vi "Are Servers Connected.vi"(5 "Wait":bool=TRUE, 6 "Activity":string, 9 "error in":errorcluster) -> (0 "Connected?":bool, 3 "error out":errorcluster)   [LabVIEW 2013]
uses:
  _ROSDefinition.vi
panel:
  out "History":string
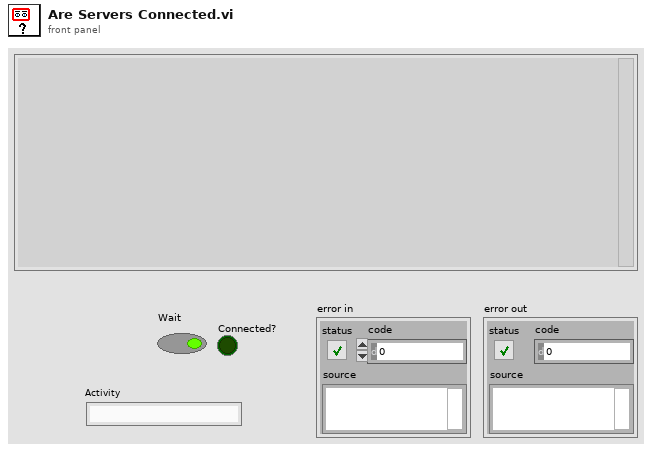
[diagram p1: front panel]
types:
  T1 = cluster{"server vi":string, "reference":refnum<vi>, "Description":string[], "Connected":bool}[]
  T2 = enum32{"Bad", "Idle", "Run top level", "Running"}
  T3 = cluster{"server vi":string, "reference":refnum<vi>, "Description":string[], "Connected":bool}
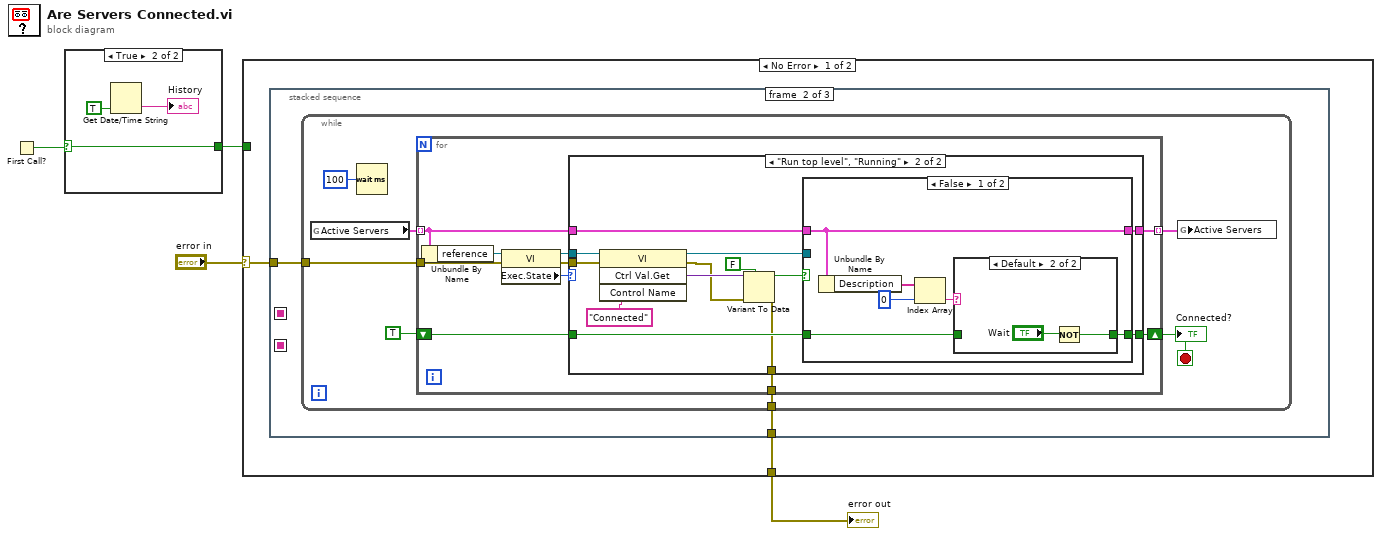
[diagram p0: block diagram]
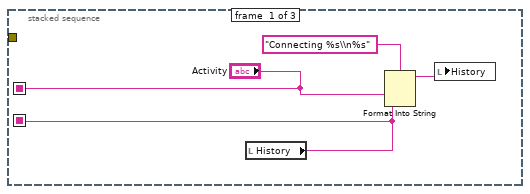
[diagram p3: hidden frame]
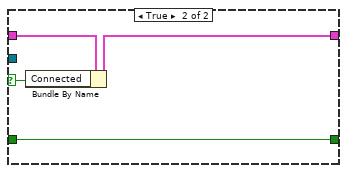
[diagram p6: hidden frame]
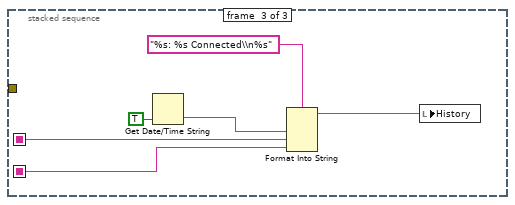
[diagram p7: hidden frame]
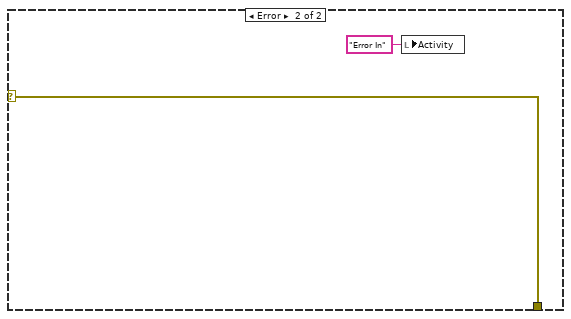
[diagram p8: hidden frame]
diagram:
  n1 = First Call?() -> (First Call?: T/F=w2:bool)
  n2 = case shown="True" w2 {
    selector: w2 -> [w5 w8]
    tunnel: [w5 w8] -> w1
    frame False {
    }
    frame True {
      n3 = Get Date/Time String(want seconds? (F)=TRUE) -> (time string=→"History":string)  [unwired: 2 in, 1 out]
    }
  }
  n4 = case shown="No Error" "error in" {
    selector: "error in" -> [w10 w70]
    tunnel: [w9 w70] -> w3
    tunnel: w1 -> [_ _]
    frame No Error {
      n5 = stacked-sequence {
        seq-local: ["Activity" _ _] -> [_ _ w65]
        seq-local: [w11 _ _] -> [_ _ w64]
        tunnel: w10 -> [_ w16 _]
        tunnel: [_ w15 _] -> w9
        frame #0 {
          n6 = local read "History"() -> (w11:string)
          n7 = Format Into String(format string="Connecting %s\\n%s", "Activity", w11) -> (resulting string=w12:string)  [unwired: 2 in, 1 out]
          n8 = local write "History"(w12) -> ()
        }
        frame #1 {
          n9 = while {
            tunnel: w16 -> [w18]
            tunnel: [w17] -> w15
            stop <- w19 stop-if-true
            n10 = global read "_ROSDefinition.vi" "Active Servers"() -> (w23:T1)
            n11 = Wait (ms)(milliseconds to wait=u32 100) -> ()  [unwired: 1 out]
            n12 = for {
              tunnel: w23 -> [w31] mode=indexing
              tunnel: [w28] -> w22 mode=indexing
              shift-right: [w26] -> w19
              shift-left: TRUE -> [w27]
              tunnel: w18 -> [w25]
              tunnel: [w24] -> w17
              n13 = Unbundle By Name(w31) -> ("reference"=w33:refnum<vi>)
              n14 = property class="VI"(reference=w33, error in=w25) -> (reference out=w30:refnum<vi>, error out=w29:errorcluster, "Exec.State"=w32:T2)
              n15 = case shown="\"Run top level\", \"Running\"" w32 {
                tunnel: w31 -> [w36 w45]
                tunnel: w30 -> [_ w49]
                tunnel: w29 -> [w34 w48]
                tunnel: [w36 w44] -> w28
                tunnel: w27 -> [w35 w40]
                tunnel: [w35 w39] -> w26
                tunnel: [w34 w37] -> w24
                frame "Bad", Default {
                }
                frame "Run top level", "Running" {
                  n16 = invoke class="VI" method="Ctrl Val.Get"(reference=w49, error in=w48, "Control Name"="Connected") -> (reference out=w43:refnum<vi>, error out=w38:errorcluster, "Get Control Value Variant"=w46:variant)  [unwired: 1 in, 1 out]
                  n17 = Variant To Data(error in=w38, type=FALSE, Variant=w46) -> (data=w41:bool, error out=w37:errorcluster)
                  n18 = case shown="False" w41 {
                    selector: w41 -> [_ w60]
                    tunnel: w45 -> [w55 w62]
                    tunnel: [w55 w61] -> w44
                    tunnel: w43 -> [_ _]
                    tunnel: w40 -> [w51 w59]
                    tunnel: [w50 w59] -> w39
                    frame False {
                      n19 = Unbundle By Name(w55) -> ("Description"=w54:string[])
                      n20 = Index Array(array=w54, index=0) -> (element=w52:string)
                      n21 = case shown="Default" w52 {
                        tunnel: w51 -> [w56 _]
                        tunnel: [w56 w57] -> w50
                        frame "/labview" {
                          # "/labview doesn't connect"
                        }
                        frame Default {
                          n22 = Not(x="Wait") -> (.not. x?=w57:bool)
                        }
                      }
                    }
                    frame True {
                      n23 = Bundle By Name(cluster=w62, "Connected"=w60) -> (w61:T3)
                    }
                  }
                }
              }
            }
            "Connected?" <- w19
            n24 = global write "_ROSDefinition.vi" "Active Servers"(w22) -> ()
          }
        }
        frame #2 {
          n25 = Get Date/Time String(want seconds? (F)=TRUE) -> (time string=w66:string)  [unwired: 2 in, 1 out]
          n26 = Format Into String(format string="%s: %s Connected\\n%s", w66, w65, w64) -> (resulting string=w67:string)  [unwired: 2 in, 1 out]
          n27 = local write "History"(w67) -> ()
        }
      }
    }
    frame Error {
      n28 = local write "Activity"("Error In" ("Activity")) -> ()
    }
  }
  "error out" <- w3
